vi "Configure Channel Ratio.vi"(0 "VISA resource name":refnum<visa-resource-name>, 1 "Scan List (Empty)":string, 5 "Enable Channel Ratio (False)":bool, 9 "Delay (0.5 sec)":dbl=0.5, 11 "error in (no error)":errorcluster) -> (4 "VISA resource name out":refnum<visa-resource-name>, 15 "error out":errorcluster)   [LabVIEW 2020, in "Keithley 27XX.lvlib"]
doc: "This VI is used to configure Channel Ratio settings.\nWith a switching module installed, the ratio of two channels can be calculated and displayed.\n\nRatio = Chan A/Chan B\nwhere: Chan A is the selected (closed) channel.\n Chan B is the paired channel for the installed switching module.\nFor example, the Model 7700 switching module has 20 channels that can use the ratio function. The primary channels (1 through 10) are linke to the paired channels (11 through 20). Channel 1 is paired to channel 11, channel 2 is paired to channel 12, and so on.\n\nNote:\n(1) The ratio calculation can only be enabled if a valid switching channel is closed.\n\n(2) A primary channel must be closed before you can enable ratio or channel average."
uses:
  Keithley 27XX.lvlib
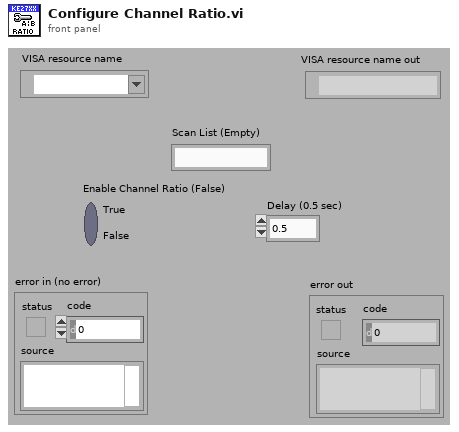
[diagram p1: front panel]
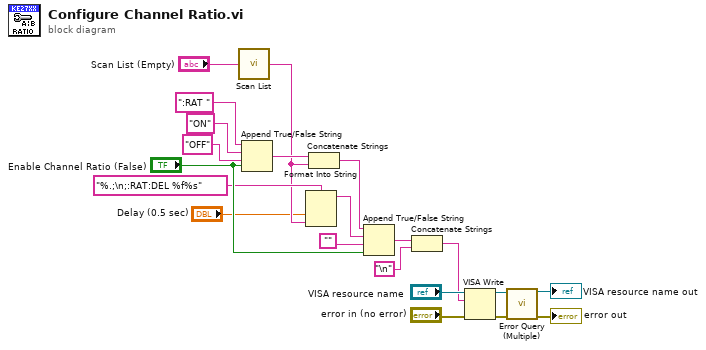
[diagram p0: block diagram]
diagram:
  n1 = call "Scan List.vi"("Scan List (Empty)"="Scan List (Empty)") -> ("Scan List Out"=w10:string)  [unwired: 14 in]
  n2 = Append True/False String(1:"Enable Channel Ratio (False)", 2:"OFF" ("string (\"\")"), 3:"ON" ("string (\"\")"), 4:":RAT " ("string (\"\")")) -> (0:w16:string)
  n3 = Format Into String(format string="%.;\n;:RAT:DEL %f%s", "Delay (0.5 sec)", w10) -> (resulting string=w8:string)  [unwired: 2 in, 1 out]
  n4 = Concatenate Strings(w16, w10) -> (w14:string)
  n5 = Append True/False String(1:"Enable Channel Ratio (False)", 2:"", 3:w8, 4:w14) -> (0:w3:string)
  n6 = Concatenate Strings(w3, "\n") -> (w1:string)
  n7 = VISA Write(VISA resource name="VISA resource name", write buffer=w1, error in (no error)="error in (no error)") -> (VISA resource name out=w7:refnum<visa-resource-name>, error out=w6:errorcluster)  [unwired: 1 out]
  n8 = call "Error Query (Multiple).vi"("VISA resource name"=w7, "error in (no error)"=w6) -> ("VISA resource name out"=→"VISA resource name out":refnum<visa-resource-name>, "error out"=→"error out":errorcluster)  [unwired: 10 in, 2 out]
